vi "Configure TV Trigger Source.vi"(0 "VISA resource name":refnum<visa-resource-name>, 1 "TV Event (0: Field 1)":u16(ring) items=["Field 1", "Field 2", "Any Field", "Any Line", "Line Number", "Vertical", "LField 1", "LField 2", "LAlternate", "LVertical"], 5 "Channel (0: Channel 1)":u16(ring) items=["Channel 1", "Channel 2", "Channel 3", "Channel 4"], 7 "TV Trigger Polarity (0: Positive)":u16(ring) items=["Positive", "Negative"], 9 "TV Signal Format (1: NTSC)":u16(ring)=1 items=["Generic", "NTSC", "PALM", "PAL", "SECAM", "P480L60HZ", "P480", "P720L60HZ", "P720", "P1080L24HZ", "P1080", "P1080L25HZ", "I1080L50HZ", "I1080", "I1080L60HZ"], 11 "error in (no error)":errorcluster, 12 "TV Line Number (1)":i32=1) -> (4 "VISA resource name out":refnum<visa-resource-name>, 15 "error out":errorcluster)   [LabVIEW 2017, in "Agilent 6000 Series.lvlib"]
doc: "This VI configures the TV trigger. You configure the TV trigger source, signal format, the event on which to trigger, and the signal polarity."
uses:
  <instrlib>/Agilent 6000 Series/Agilent 6000 Series.lvlib
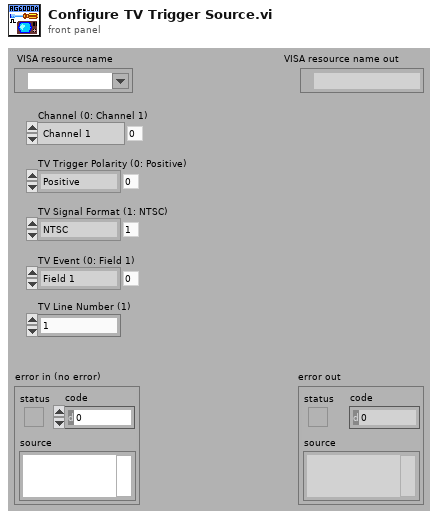
[diagram p1: front panel]
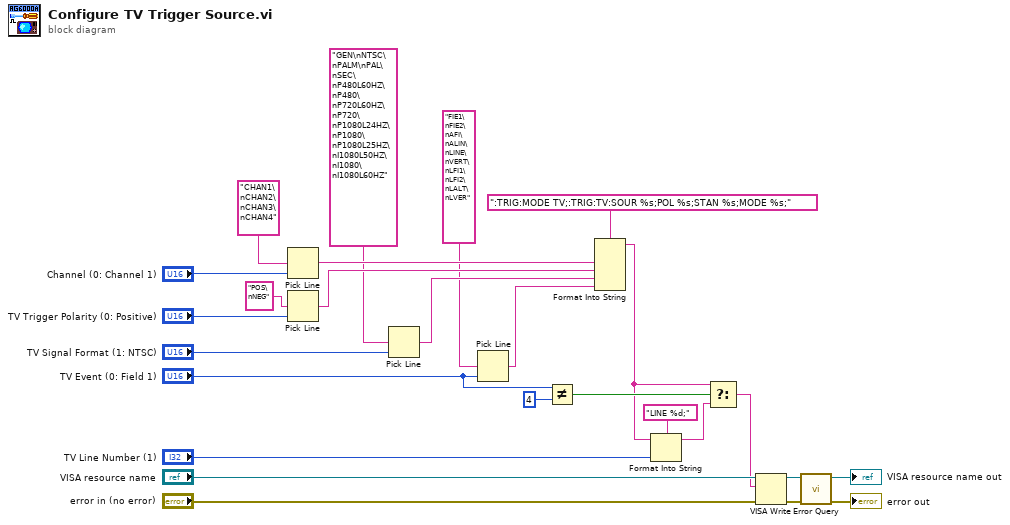
[diagram p0: block diagram]
diagram:
  n1 = Pick Line(multi-line string="CHAN1\nCHAN2\nCHAN3\nCHAN4", line index="Channel (0: Channel 1)") -> (output string=w19:string)  [unwired: 1 in]
  n2 = Pick Line(multi-line string="POS\nNEG", line index="TV Trigger Polarity (0: Positive)") -> (output string=w17:string)  [unwired: 1 in]
  n3 = Pick Line(multi-line string="GEN\nNTSC\nPALM\nPAL\nSEC\nP480L60HZ\nP480\nP720L60HZ\nP720\nP1080L24HZ\nP1080\nP1080L25HZ\nI1080L50HZ\nI1080\nI1080L60HZ", line index="TV Signal Format (1: NTSC)") -> (output string=w15:string)  [unwired: 1 in]
  n4 = Pick Line(multi-line string="FIE1\nFIE2\nAFI\nALIN\nLINE\nVERT\nLFI1\nLFI2\nLALT\nLVER", line index="TV Event (0: Field 1)") -> (output string=w13:string)  [unwired: 1 in]
  n5 = Not Equal?(x="TV Event (0: Field 1)", y=u16 4) -> (x != y?=w6:bool)
  n6 = Format Into String(format string=":TRIG:MODE TV;:TRIG:TV:SOUR %s;POL %s;STAN %s;MODE %s;" ("Source Command"), w19, w17, w15, w13) -> (resulting string=w4:string)  [unwired: 2 in, 1 out]
  n7 = Format Into String(format string="LINE %d;", initial string=w4, "TV Line Number (1)") -> (resulting string=w2:string)  [unwired: 1 in, 1 out]
  n8 = Select(t=w4, s=w6, f=w2) -> (s? t:f=w1:string)
  n9 = VISA Write(VISA resource name="VISA resource name", write buffer=w1, error in (no error)="error in (no error)") -> (VISA resource name out=w22:refnum<visa-resource-name>, error out=w21:errorcluster)  [unwired: 1 out]
  n10 = call <instrlib>:"Error Query.vi"("error in (no error)"=w21, "VISA resource name"=w22) -> ("error out"=→"error out":errorcluster, "VISA resource name out"=→"VISA resource name out":refnum<visa-resource-name>)  [unwired: 6 in, 2 out]
